vi "Periodic Tasks.vi"(8 "error in":errorcluster) -> ()   [LabVIEW 2017]
doc: "This VI runs in parallel to other tasks. It can contain as many user-defined periodic loops as you need. These can carry out PID or other sorts of timed response."
uses:
  <vilib>/Rock Robotics/WPI/DriverStation/WPI_DriverStationRobotMode2.ctl
  <vilib>/Rock Robotics/WPI/Utilities/WPI_GetSetVariantRefNum.vi
  Robot Global Data.vi
  <vilib>/Rock Robotics/WPI/ThirdParty/Phoenix-LabVIEW/Pigeon IMU/CTRE_PigeonIMU_GetYPR.vi
panel:
  out "Gyro Yaw Out":dbl=-0.1318359375 format="%#_13g"
  out "Drive Loop Speed":u32=24
  in  "Drive wait":u32=25
  in  "Joystick wait":u32=25
  out "Joystick Loop Speed":u32=24
  in  "Rot Pt X":dbl format="%#_13g"
  in  "Rot Pt Y":dbl format="%#_13g"
  out "Robot Centric?":bool
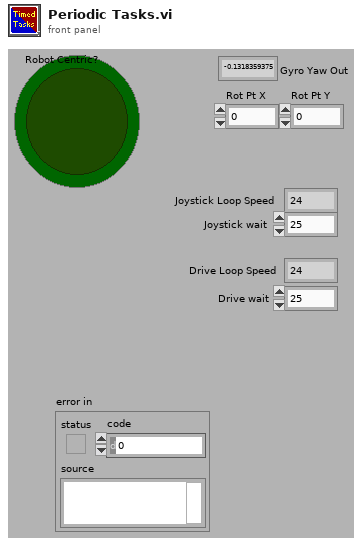
[diagram p1: front panel]
types:
  T1 = typedef "WPI_JoystickDevRef.ctl" = cluster{"Device":T2}
  T2 = typedef "WPI_JoystickDeviceEnum.ctl" = enum16{"USB 0", "USB 1", "USB 2", "USB 3", "USB 4", "USB 5"}
  T3 = typedef "WPI_DriverStationRobotMode2.ctl" = enum16{"Autonomous Disabled", "Autonomous Enabled", "Teleop Disabled", "Teleop Enabled", "Disconnected", "Finish", "Test Disabled", "Test Enabled", "Emergency Stopped"}
  T4 = typedef "CTRE_PigeonIMU_DeviceRef.ctl" = cluster{"DeviceStatus":errorcluster, "Device Number":u8, "Type":T5, "Device ID":u32, "Handle":u64, "UsageFrame":u32, "Library Path":path}
  T5 = typedef "CTRE_PigeonIMU_ConnectionType.ctl" = u32
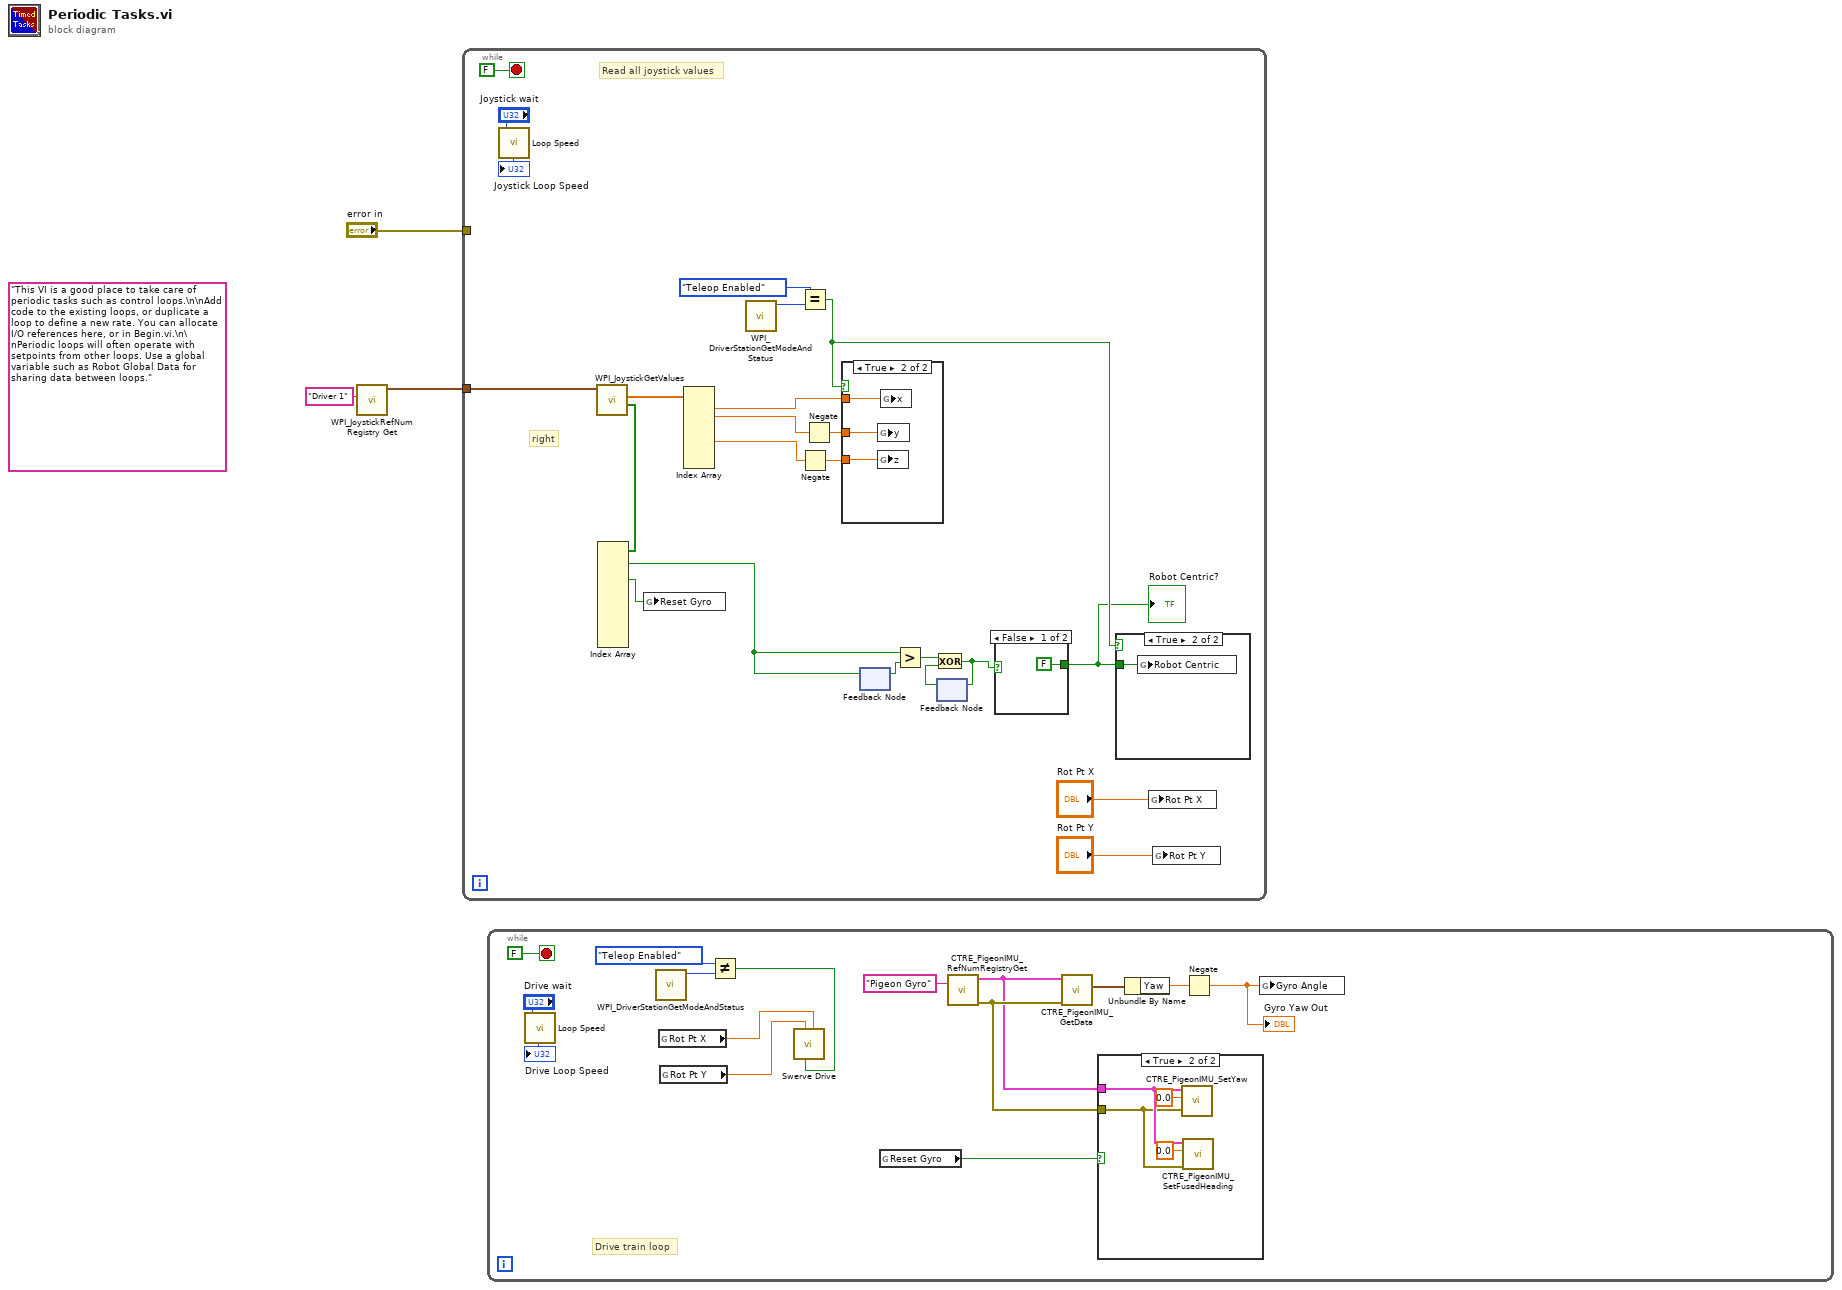
[diagram p0: block diagram]
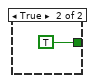
[diagram p3: hidden frame]
diagram:
  (unwired) "This VI is a good place to take care of periodic tasks such as control loops.\n\nAdd code to the existing loops, or duplicate a loop to define a new rate. You can allocate I/O references here, or in Begin.vi.\n\nPeriodic loops will often operate with setpoints from other loops. Use a global variable such as Robot Global Data for sharing data between loops."
  n1 = call <vilib>:"WPI_JoystickRefNum Registry Get.vi"("refnum name"="Driver 1") -> ("JoystickDevRef"=w2:T1)  [unwired: 9 in, 1 out]
  n2 = while {
    tunnel: w2 -> [w21]
    tunnel: "error in" -> [_]
    stop <- FALSE stop-if-true
    # "Read all joystick values"
    # "right"
    n3 = call "Loop Speed.vi"("milliseconds to wait"="Joystick wait") -> ("Loop Speed"=→"Joystick Loop Speed":u32)
    n4 = call <vilib>:"WPI_JoystickGetValues.vi"("JoystickDevRef"=w21) -> ("Buttons"=w24:bool[], "Axes"=w25:dbl[])  [unwired: 6 in, 3 out]
    n5 = Index Array(array=w24) -> (element #1=w8:bool, element #3=w12:bool)  [unwired: 11 in, 9 out]
    n6 = global write "Robot Global Data.vi" "Reset Gyro"(w12) -> ()
    n7 = Index Array(array=w25) -> (element #1=w23:dbl, element #2=w22:dbl, element #5=w13:dbl)  [unwired: 8 in, 5 out]
    n8 = call <vilib>:"WPI_DriverStationGetModeAndStatus.vi"() -> ("Robot Mode"=w20:T3)  [unwired: 10 in, 1 out]
    n9 = Equal?(x=WPI_DriverStationRobotMode2."Teleop Enabled", y=w20) -> (x = y?=w18:bool)
    n10 = Negate(x=w13) -> (-x=w4:dbl)
    n11 = Negate(x=w22) -> (-x=w5:dbl)
    n12 = case shown="True" w18 {
      tunnel: w5 -> [_ w31]
      tunnel: w23 -> [_ w32]
      tunnel: w4 -> [_ w30]
      frame False {
      }
      frame True {
        n13 = global write "Robot Global Data.vi" "y"(w31) -> ()
        n14 = global write "Robot Global Data.vi" "z"(w30) -> ()
        n15 = global write "Robot Global Data.vi" "x"(w32) -> ()
      }
    }
    n16 = feedback #1() -> (w11:bool)  [unwired: 1 in]
    n17 = feedback-in #1(w8) -> ()
    n18 = Greater?(x=w8, y=w11) -> (0:w10:bool)
    n19 = feedback #2() -> (w9:bool)  [unwired: 1 in]
    n20 = Exclusive Or(1:w9, 2:w10) -> (0:w6:bool)
    n21 = feedback-in #2(w6) -> ()
    n22 = case shown="False" w6 {
      tunnel: [FALSE TRUE] -> w7
      frame False {
      }
      frame True {
      }
    }
    "Robot Centric?" <- w7
    n23 = case shown="True" w18 {
      tunnel: w7 -> [_ w29]
      frame False {
      }
      frame True {
        n24 = global write "Robot Global Data.vi" "Robot Centric"(w29) -> ()
      }
    }
    n25 = global write "Robot Global Data.vi" "Rot Pt X"("Rot Pt X") -> ()
    n26 = global write "Robot Global Data.vi" "Rot Pt Y"("Rot Pt Y") -> ()
  }
  n27 = while {
    stop <- FALSE stop-if-true
    # "Drive train loop"
    n28 = call "Loop Speed.vi"("milliseconds to wait"="Drive wait") -> ("Loop Speed"=→"Drive Loop Speed":u32)
    n29 = call <vilib>:"WPI_DriverStationGetModeAndStatus.vi"() -> ("Robot Mode"=w45:T3)  [unwired: 10 in, 1 out]
    n30 = global read "Robot Global Data.vi" "Rot Pt X"() -> (w36:dbl)
    n31 = global read "Robot Global Data.vi" "Rot Pt Y"() -> (w37:dbl)
    n32 = Not Equal?(x=WPI_DriverStationRobotMode2."Teleop Enabled", y=w45) -> (x != y?=w35:bool)
    n33 = call "Swerve Drive.vi"("Rot. Point X"=w36, "Auto Controls"=w35, "Rot. Point Y"=w37) -> ()  [unwired: 9 in]
    n34 = global read "Robot Global Data.vi" "Reset Gyro"() -> (w40:bool)
    n35 = call <vilib>:"CTRE_PigeonIMU_RefNumRegistryGet.vi"("refnum name"="Pigeon Gyro") -> ("error out"=w42:errorcluster, "PigeonIMUDevRef"=w41:T4)  [unwired: 9 in]
    n36 = call-poly <vilib>:"CTRE_PigeonIMU_GetData.vi"("error in (no error)"=w42, "PigeonIMUDevRef"=w41) -> ("Yaw Pitch Roll"=w39:cluster{"Yaw":dbl, "Pitch":dbl, "Roll":dbl})  [unwired: 7 in, 2 out]
    n37 = case shown="True" w40 {
      tunnel: w41 -> [_ w49]
      tunnel: w42 -> [_ w48]
      frame False {
      }
      frame True {
        n38 = call <vilib>:"CTRE_PigeonIMU_SetYaw.vi"("error in (no error)"=w48, "Value"=0.0, "PigeonIMUDevRef"=w49) -> ()  [unwired: 7 in, 2 out]
        n39 = call <vilib>:"CTRE_PigeonIMU_SetFusedHeading.vi"("error in (no error)"=w48, "Value"=0.0, "PigeonIMUDevRef 2"=w49) -> ()  [unwired: 7 in, 2 out]
      }
    }
    n40 = Unbundle By Name(w39) -> ("Yaw"=w43:dbl)
    n41 = Negate(x=w43) -> (-x=w33:dbl)
    "Gyro Yaw Out" <- w33
    n42 = global write "Robot Global Data.vi" "Gyro Angle"(w33) -> ()
  }
